vi "Version Scripting.vi"(9 "Project":refnum<vi>, 10 "To":T1, 11 "From":T1) -> ()   [LabVIEW 2020]
uses:
  Version.ctl
  Tags.ctl
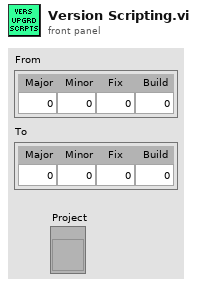
[diagram p1: front panel]
types:
  T1 = typedef "Version.ctl" = cluster{"Major":u16, "Minor":u16, "Fix":u16, "Build":u16}
  T2 = typedef "Tags.ctl" = enum16{"sol.formulag.version"}
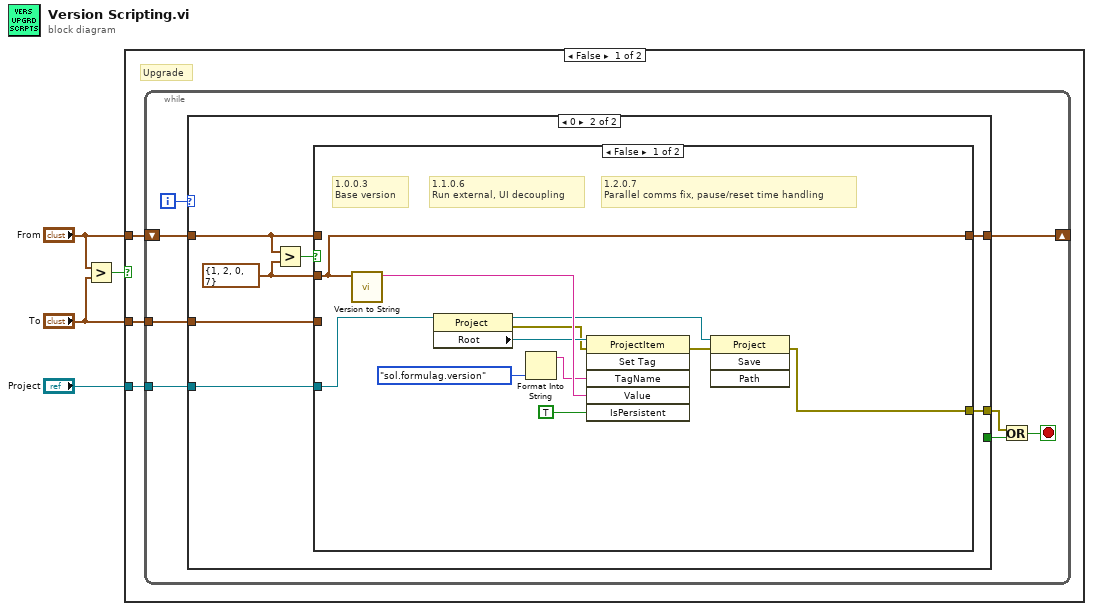
[diagram p0: block diagram]
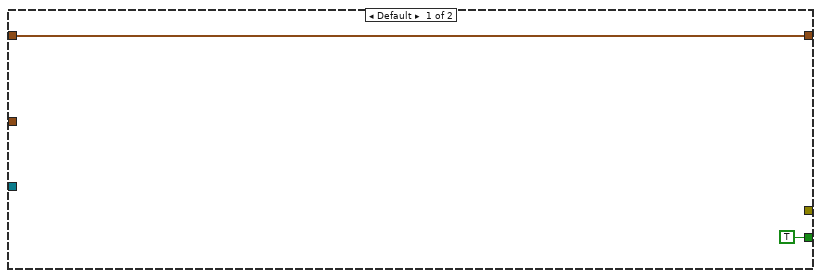
[diagram p2: hidden frame]
diagram:
  n1 = Greater?(x="From", y="To") -> (0:w1:bool)
  n2 = case shown="False" w1 {
    tunnel: "Project" -> [w7 _]
    tunnel: "From" -> [w6 _]
    tunnel: "To" -> [w5 _]
    frame False {
      # "Upgrade"
      n3 = while {
        shift-right: [w13] -> _
        shift-left: w6 -> [w14]
        tunnel: w7 -> [w10]
        tunnel: w5 -> [w12]
        i -> [w15]
        stop <- w9 stop-if-true
        n4 = case shown="0" w15 {
          tunnel: w14 -> [w16 w22]
          tunnel: [w16 w21] -> w13
          tunnel: w12 -> [_ w20]
          tunnel: [TRUE _] -> w11
          tunnel: w10 -> [_ w19]
          tunnel: [_ w18] -> w8
          frame Default {
          }
          frame 0 {
            w23 = T1 {"Major"=1, "Minor"=2, "Fix"=0, "Build"=7} ("y")
            n5 = Greater?(x=w22, y=w23) -> (0:w24:bool)
            n6 = case shown="False" w24 {
              tunnel: w23 -> [w35 _]
              tunnel: w22 -> [_ w36]
              tunnel: [w35 w36] -> w21
              tunnel: w20 -> [_ _]
              tunnel: w19 -> [w32 _]
              tunnel: [w34 _] -> w18
              frame False {
                # "1.2.0.7\nParallel comms fix, pause/reset time handling"
                # "1.1.0.6\nRun external, UI decoupling"
                # "1.0.0.3\nBase version"
                n7 = call "Version to String.vi"("Version"=w35) -> ("Version String"=w33:string)  [unwired: 10 in]
                n8 = property class="Project"(reference=w32) -> (reference out=w26:refnum<vi>, error out=w27:errorcluster, "Root"=w31:refnum<vi>)  [unwired: 1 in]
                n9 = Format Into String(Tags."sol.formulag.version" ("Tags")) -> (resulting string=w29:string)  [unwired: 3 in, 1 out]
                n10 = invoke class="ProjectItem" method="Set Tag"(reference=w31, error in=w27, "TagName"=w29, "Value"=w33, "IsPersistent"=TRUE ("Is Persistent (T)")) -> (error out=w25:errorcluster)  [unwired: 1 in, 5 out]
                n11 = invoke class="Project" method="Save"(reference=w26, error in=w25) -> (error out=w34:errorcluster)  [unwired: 2 in, 3 out]
              }
              frame True {
                # "Already greater than 1.0.0.3, nothing to do for this step."
              }
            }
          }
        }
        n12 = Or(x=w8, y=w11) -> (x .or. y?=w9:bool)
      }
    }
    frame True {
      # "Downgrade"
    }
  }
